vi "Save Trip File.vi"(8 "error in":errorcluster, 11 "FPGA Refnum":T1) -> (0 "Error Out":errorcluster)   [LabVIEW 2020]
doc: "Author: Scott Hannahs <sth@magnet.fsu.edu>\nCopyright 2018 Florida State University, All rights reserved."
uses:
  RT Controls/FPGA SCH Digitizer Ref.ctl
  RT Host Globals.vi
  <vilib>/regexp/Match Regular Expression.xnode
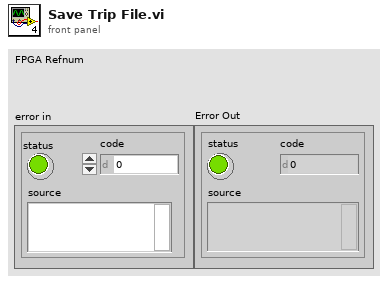
[diagram p1: front panel]
types:
  T1 = typedef "FPGA SCH Digitizer Ref.ctl" = refnum<k20>
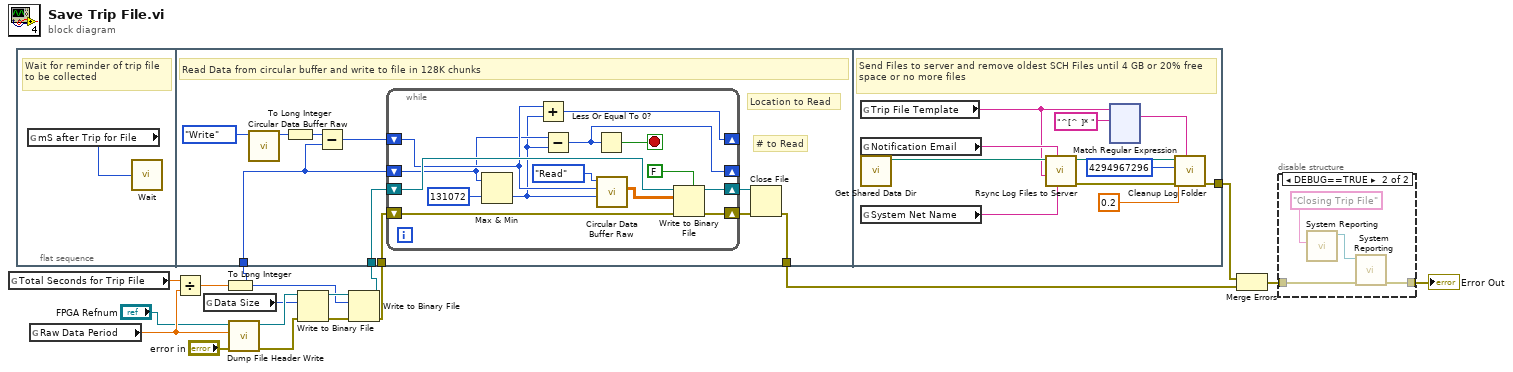
[diagram p0: block diagram]
diagram:
  n1 = global read "RT Host Globals.vi" "Total Seconds for Trip File"() -> (w8:dbl)
  n2 = flat-sequence {
    tunnel: w11 -> [w23]
    tunnel: w10 -> [w22]
    tunnel: w9 -> [w21]
    tunnel: [w19] -> w4
    tunnel: [w52] -> w5
    frame #0 {
      # "Wait for reminder of trip file to be collected"
      n3 = global read "RT Host Globals.vi" "mS after Trip for File"() -> (w18:u32)
      n4 = call "Wait"("Count(mSec)"=w18) -> ()  [unwired: 1 out]
    }
    frame #1 {
      # "Location to Read"
      # "# to Read"
      # "Read Data from circular buffer and write to file in 128K chunks"
      n5 = call "Circular Data Buffer Raw.vi"("Enum"=enum16{"Initialize", "Write", "Read"}."Write") -> ("Next Write"=w27:u32)  [unwired: 8 in, 2 out]
      n6 = To Long Integer(number=w27) -> (32bit integer=w28:i32)
      n7 = Subtract(x=w28, y=w23) -> (x-y=w20:i32)
      n8 = while {
        shift-right: [w29] -> _
        shift-left: w20 -> [w35]
        shift-right: [w30] -> _
        shift-left: w23 -> [w34]
        shift-right: [w38] -> w25
        shift-left: w22 -> [w40]
        shift-right: [w37] -> w24
        shift-left: w21 -> [w39]
        stop <- w31 stop-if-true
        n9 = Max & Min(x=w34, y=131072 ("x")) -> (min(x,y)=w32:i32)  [unwired: 1 out]
        n10 = Add(x=w35, y=w32) -> (x+y=w29:i32)
        n11 = Subtract(x=w34, y=w32) -> (x-y=w30:i32)
        n12 = Less Or Equal To 0?(x=w30) -> (x <= 0?=w31:bool)
        n13 = call "Circular Data Buffer Raw.vi"("Read Size"=w32, "Read Location"=w35, "Enum"=enum16{"Initialize", "Write", "Read"}."Read") -> ("Data Out"=w41:dbl[][])  [unwired: 6 in, 2 out]
        n14 = Write to Binary File(file (use dialog)=w40, data=w41, error in=w39, 5:FALSE ("prepend array or string size? (T)")) -> (refnum out=w38:refnum<file>, error out=w37:errorcluster)  [unwired: 2 in, 1 out]
      }
      n15 = Close File(refnum=w25, error in=w24) -> (error out=w19:errorcluster)  [unwired: 1 out]
    }
    frame #2 {
      # "Send Files to server and remove oldest SCH Files until 4 GB or 20% free space or no more files"
      n16 = global read "RT Host Globals.vi" "Trip File Template"() -> (w45:string)
      n17 = global read "RT Host Globals.vi" "Notification Email"() -> (w47:string)
      n18 = call "Get Shared Data Dir.vi"() -> ("Data Directory Path"=w48:path)  [unwired: 2 in, 1 out]
      n19 = global read "RT Host Globals.vi" "System Net Name"() -> (w46:string)
      n20 = call "Rsync Log Files to Server.vi"("System Net Name"=w46, "Recipients"=w47, "Log File Template"=w45, "Log File Path In"=w48) -> ("Error Out"=w50:errorcluster, "Log File Path Out"=w53:path)  [unwired: 3 in, 3 out]
      n21 = xnode "Match Regular Expression"("input string"=w45, "regular expression"="^[^ ]* ") -> ("whole match"=w43:string)  [unwired: 4 in, 4 out]
      n22 = call "Cleanup Log Folder.vi"("Template"=w43, "Error In"=w50, "Min Fraction"=0.2, "Min Space"=i64 4294967296 ("y"), "Log File Path In"=w53) -> ("Error Out"=w52:errorcluster)  [unwired: 6 in]
    }
  }
  n23 = global read "RT Host Globals.vi" "Raw Data Period"() -> (w7:dbl)
  n24 = Divide(x=w8, y=w7) -> (x/y=w17:dbl)
  n25 = global read "RT Host Globals.vi" "Data Size"() -> (w14:u32)
  n26 = To Long Integer(number=w17) -> (32bit integer=w11:i32)
  n27 = call "Dump File Header Write.vi"("error in"="error in", "Raw Data Period"=w7, "FPGA Refnum"="FPGA Refnum") -> ("error out"=w16:errorcluster, "Byte Stream File out"=w15:refnum<file>)  [unwired: 6 in, 1 out]
  n28 = Write to Binary File(file (use dialog)=w15, data=w14, error in=w16) -> (refnum out=w12:refnum<file>, error out=w13:errorcluster)  [unwired: 3 in, 1 out]
  n29 = Write to Binary File(file (use dialog)=w12, data=w11, error in=w13) -> (refnum out=w10:refnum<file>, error out=w9:errorcluster)  [unwired: 3 in, 1 out]
  n30 = Merge Errors(w5, w4) -> (w2:errorcluster)
  n31 = disable-structure shown="DEBUG==TRUE" {
    disable-tunnel: w2 -> [w168 w170]
    disable-tunnel: [w168 w169] -> w1
    frame condition #0 (active) {
    }
    frame condition #1 {
      n32 = call "System Reporting.vi"("String"="Closing Trip File") -> ("Byte Stream File out"=w172:refnum<file>)  [unwired: 9 in, 1 out]
      n33 = call "System Reporting.vi"("Error In"=w170, "Byte Stream File in"=w172) -> ("Error Out"=w169:errorcluster)  [unwired: 8 in, 1 out]
    }
  }
  "Error Out" <- w1
